vi "tikki.vi"   [LabVIEW 2016]
uses:
  <vilib>/NXT/Subs/LVHSConnector.ctl
  <vilib>/NXT/LegoClasses/BrickReference/BrickReference.lvclass
  <vilib>/NXT/Block Support/NXT_OutputPort.ctl
  <vilib>/NXT/Block Support/NXT_ButtonSelector.ctl
  <vilib>/NXT/Block Support/NXT_InputPort.ctl
  <vilib>/NXT/Dual Mode Library/Waits/Wait_Num.vi
  <vilib>/NXT/NXTIO Xnodes/NXTIONodeSubVIs/NXTMoveMotors.vi
  <vilib>/NXT/Dual Mode Library/Sensors/EV3_Color_Reflect.vi
  <vilib>/NXT/Dual Mode Library/Sound/PlayB.vi
  <vilib>/NXT/Dual Mode Library/Sensors/EV3_Ultrasonic_CM.vi
  <vilib>/NXT/Dual Mode Library/Sensors/readNXTButton.vi
  <vilib>/NXT/NXTIO Xnodes/AddressXNode/NXTIOAddress.xnode
  <vilib>/NXT/NXTIO Xnodes/NXTIOXNode/NXTIO.xnode
types:
  T1 = typedef "LVHSConnector.ctl" = refnum<class "BrickReference.lvclass">
  T2 = typedef "NXT_OutputPort.ctl" = u8
  T3 = typedef "NXT_InputPort.ctl" = u32
  T4 = typedef "NXT_ButtonSelector.ctl" = u16
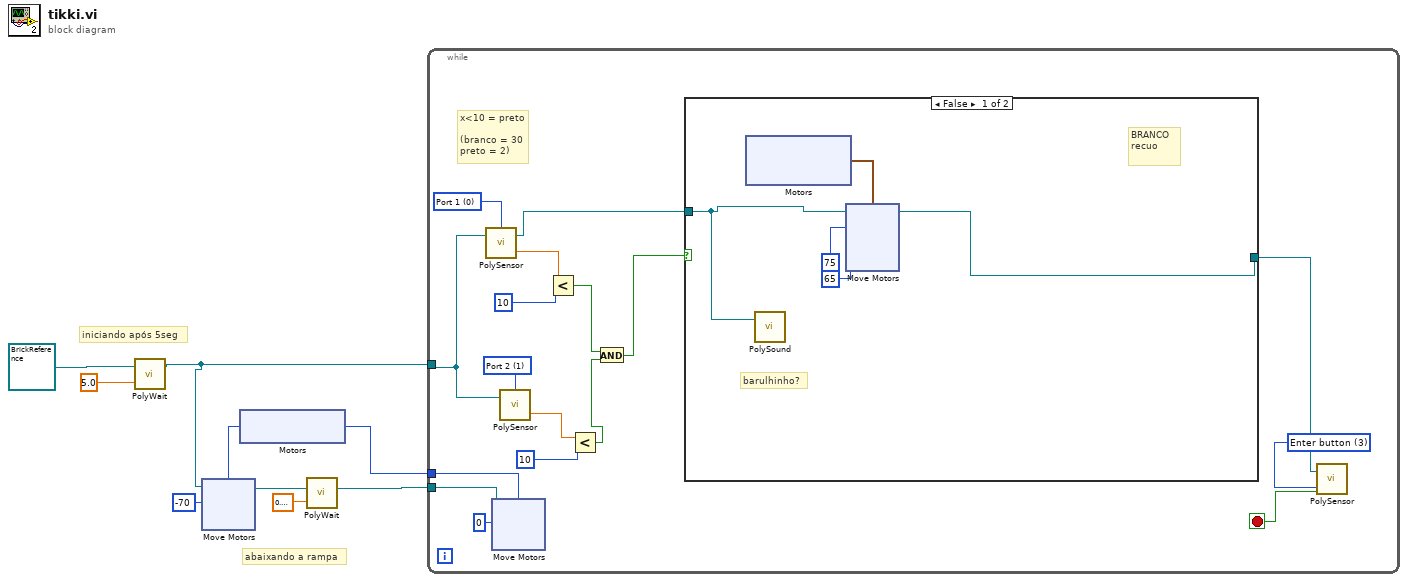
[diagram p0: block diagram]
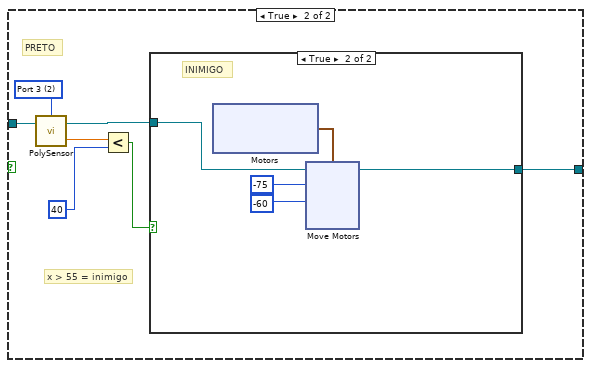
[diagram p2: hidden frame]
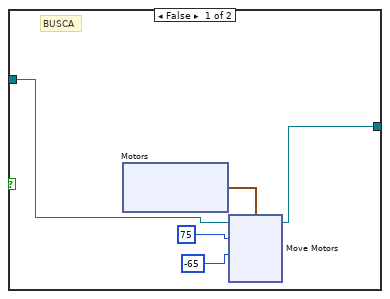
[diagram p3: hidden frame]
diagram:
  # "iniciando após 5seg"
  # "abaixando a rampa"
  n1 = call-poly <vilib>:"PolyWait.vi"("Time (1 sec)"=sgl 5.0, "NXT/EV3"=T1 refnum) -> ("NXT/EV3"=w3:T1)  [unwired: 2 in]
  n2 = xnode "Motors"() -> ("Motor"=w2:T2)
  n3 = xnode "Move Motors"("Power/Speed 1"=i8 -70, "Motors"=w2, "NXT/EV3"=w3) -> ("NXT/EV3"=w6:T1)
  n4 = call-poly <vilib>:"PolyWait.vi"("Time (1 sec)"=sgl 0.3, "NXT/EV3"=w6) -> ("NXT/EV3"=w1:T1)  [unwired: 2 in]
  n5 = while {
    tunnel: w3 -> [w20]
    tunnel: w2 -> [w11]
    tunnel: w1 -> [w10]
    stop <- w25 stop-if-true
    w12 = T3 1 items=["Port 1", "Port 2", "Port 3", "Port 4"] ("Port (Port 1)")
    w13 = T3 0 items=["Port 1", "Port 2", "Port 3", "Port 4"] ("Port (Port 1)")
    w24 = T4 3 items=["Enter button"=3, "Left button"=2, "Right button"=1, "Up Button"=4, "Down Button"=5] ("Button (Enter button)")
    # "x<10 = preto\n\n(branco = 30\npreto = 2)"
    n6 = call-poly <vilib>:"PolySensor.vi"("NXT/EV3"=w20, "Port (Port 1)"=w13) -> ("Scaled Value"=w23:sgl, "NXT/EV3"=w14:T1)  [unwired: 1 in]
    n7 = xnode "Move Motors"("Power/Speed 1"=i8 0, "Motors"=w11, "NXT/EV3"=w10) -> ()  [unwired: 1 out]
    n8 = call-poly <vilib>:"PolySensor.vi"("NXT/EV3"=w20, "Port (Port 1)"=w12) -> ("Scaled Value"=w18:sgl)  [unwired: 1 in, 1 out]
    n9 = Less?(x=w23, y=10) -> (x < y?=w17:bool)
    n10 = Less?(x=w18, y=10) -> (x < y?=w16:bool)
    n11 = And(x=w17, y=w16) -> (x .and. y?=w15:bool)
    n12 = case shown="False" w15 {
      tunnel: [w33 w49] -> w22
      tunnel: w14 -> [w34 w48]
      frame False {
        # "barulhinho?"
        # "BRANCO\nrecuo"
        n13 = xnode "Motors"() -> ("Motor"=w36:cluster{"Port":T2, "Port":T2})
        n14 = call-poly <vilib>:"PolySound.vi"("NXT/EV3"=w34) -> ()  [unwired: 3 in, 1 out]
        n15 = xnode "Move Motors"("Power/Speed 2"=i8 65, "Power/Speed 1"=i8 75, "Motors"=w36, "NXT/EV3"=w34) -> ("NXT/EV3"=w33:T1)
      }
      frame True {
        w47 = T3 2 items=["Port 1", "Port 2", "Port 3", "Port 4"] ("Port (Port 1)")
        # "PRETO"
        # "x > 55 = inimigo"
        n16 = call-poly <vilib>:"PolySensor.vi"("NXT/EV3"=w48, "Port (Port 1)"=w47) -> ("Centimeters"=w53:sgl, "NXT/EV3"=w50:T1)  [unwired: 1 in]
        n17 = Less?(x=w53, y=40) -> (x < y?=w51:bool)
        n18 = case shown="True" w51 {
          tunnel: w50 -> [w54 w71]
          tunnel: [w58 w70] -> w49
          frame False {
            # "BUSCA"
            n19 = xnode "Motors"() -> ("Motor"=w57:cluster{"Port":T2, "Port":T2})
            n20 = xnode "Move Motors"("Power/Speed 2"=i8 -65, "Power/Speed 1"=i8 75, "Motors"=w57, "NXT/EV3"=w54) -> ("NXT/EV3"=w58:T1)
          }
          frame True {
            # "INIMIGO"
            n21 = xnode "Motors"() -> ("Motor"=w69:cluster{"Port":T2, "Port":T2})
            n22 = xnode "Move Motors"("Power/Speed 2"=i8 -60, "Power/Speed 1"=i8 -75, "Motors"=w69, "NXT/EV3"=w71) -> ("NXT/EV3"=w70:T1)
          }
        }
      }
    }
    n23 = call-poly <vilib>:"PolySensor.vi"("Button (Enter button)"=w24, "NXT/EV3"=w22) -> ("Yes/No"=w25:bool)  [unwired: 1 in, 1 out]
  }
